vi "CPT Delta_leakage_mlpm 12.1.vi"(1 "IN Pore":dbl, 3 "IN Side":dbl, 5 "IN Axial":dbl, 9 "Reset":bool) -> (11 "Time Out":dbl, 15 "OUT Pore Leakage":dbl, 17 "OUT Side Leakage":dbl, 19 "OUT Axial Leakage":dbl)   [LabVIEW 2015]
panel:
  out "ml Save Axial Leakage":dbl
  out "ml Save Axial":dbl
  out "ml Save Side Leakage":dbl
  out "ml Save Side":dbl
  out "ml Save Pore Leakage":dbl
  in  "seconds to wait":dbl=60.0
  out "Index":dbl
  out "millisecond timer value":u32
  out "ml Save Pore":dbl
  out "Time Save":u32
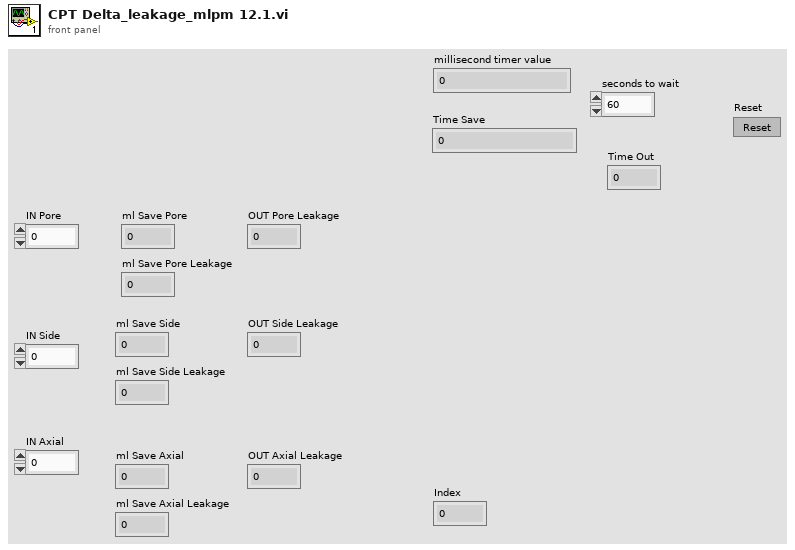
[diagram p1: front panel]
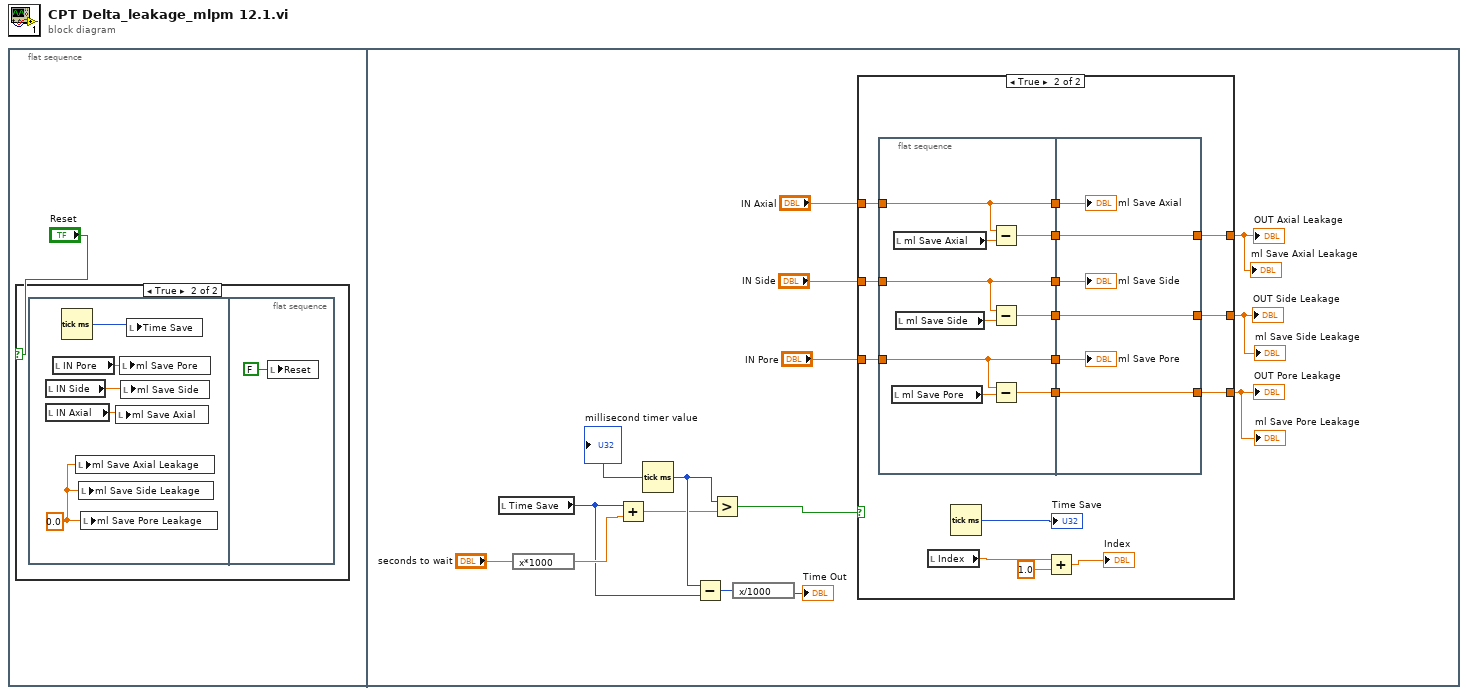
[diagram p0: block diagram]
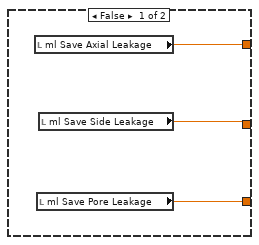
[diagram p3: hidden frame]
diagram:
  n1 = flat-sequence {
    frame #0 {
      n2 = case shown="True" "Reset" {
        frame False {
        }
        frame True {
          n3 = flat-sequence {
            frame #0 {
              w5 = 0.0 ("ml Save Pore Leakage")
              n4 = local read "IN Side"() -> (w2:dbl)
              n5 = local read "IN Axial"() -> (w3:dbl)
              n6 = local read "IN Pore"() -> (w4:dbl)
              n7 = Tick Count (ms)() -> (millisecond timer value=w6:u32)
              n8 = local write "ml Save Axial Leakage"(w5) -> ()
              n9 = local write "ml Save Side Leakage"(w5) -> ()
              n10 = local write "ml Save Pore Leakage"(w5) -> ()
              n11 = local write "ml Save Axial"(w3) -> ()
              n12 = local write "ml Save Pore"(w4) -> ()
              n13 = local write "ml Save Side"(w2) -> ()
              n14 = local write "Time Save"(w6) -> ()
            }
            frame #1 {
              n15 = local write "Reset"(FALSE ("Reset")) -> ()
            }
          }
        }
      }
    }
    frame #1 {
      n16 = local read "Time Save"() -> (w8:u32)
      n17 = expression code="x*1000"("seconds to wait") -> (w15:dbl)
      n18 = Add(x=w8, y=w15) -> (x+y=w18:dbl)
      n19 = Tick Count (ms)() -> (millisecond timer value=w19:u32)
      "millisecond timer value" <- w19
      n20 = Subtract(x=w19, y=w8) -> (x-y=w14:u32)
      n21 = Greater?(x=w19, y=w18) -> (0:w21:bool)
      n22 = expression code="x/1000"(w14) -> (→"Time Out":u32)
      n23 = case shown="True" w21 {
        tunnel: "IN Pore" -> [_ w38]
        tunnel: [w24 w33] -> w13
        tunnel: "IN Axial" -> [_ w32]
        tunnel: "IN Side" -> [_ w31]
        tunnel: [w22 w26] -> w10
        tunnel: [w23 w25] -> w9
        frame False {
          n24 = local read "ml Save Axial Leakage"() -> (w22:dbl)
          n25 = local read "ml Save Pore Leakage"() -> (w24:dbl)
          n26 = local read "ml Save Side Leakage"() -> (w23:dbl)
        }
        frame True {
          n27 = flat-sequence {
            tunnel: [w49] -> w39
            tunnel: w38 -> [w49]
            tunnel: [w47] -> w34
            tunnel: w32 -> [w42]
            tunnel: w31 -> [w45]
            tunnel: [w42] -> w30
            tunnel: [w45] -> w29
            tunnel: [w44] -> w28
            tunnel: [w43] -> w27
            tunnel: w39 -> [w55]
            tunnel: w34 -> [w54]
            tunnel: [w54] -> w33
            tunnel: w30 -> [w53]
            tunnel: w29 -> [w52]
            tunnel: [w51] -> w25
            tunnel: w28 -> [w51]
            tunnel: [w50] -> w26
            tunnel: w27 -> [w50]
            frame #0 {
              n28 = local read "ml Save Pore"() -> (w48:dbl)
              n29 = local read "ml Save Axial"() -> (w41:dbl)
              n30 = local read "ml Save Side"() -> (w46:dbl)
              n31 = Subtract(x=w42, y=w41) -> (x-y=w43:dbl)
              n32 = Subtract(x=w45, y=w46) -> (x-y=w44:dbl)
              n33 = Subtract(x=w49, y=w48) -> (x-y=w47:dbl)
            }
            frame #1 {
              "ml Save Pore" <- w55
              "ml Save Axial" <- w53
              "ml Save Side" <- w52
            }
          }
          n34 = local read "Index"() -> (w37:dbl)
          n35 = Tick Count (ms)() -> (millisecond timer value=→"Time Save":u32)
          n36 = Add(x=w37, y=1.0) -> (x+y=→"Index":dbl)
        }
      }
      "OUT Pore Leakage" <- w13
      "ml Save Pore Leakage" <- w13
      "OUT Axial Leakage" <- w10
      "OUT Side Leakage" <- w9
      "ml Save Axial Leakage" <- w10
      "ml Save Side Leakage" <- w9
    }
  }
